vi "TalonFXSet.vi"   [LabVIEW 2023]
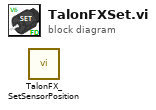
[diagram p0: block diagram]
diagram:
  n1 = call <vilib>:"TalonFX_SetSensorPosition.vi"() -> ()  [unwired: 11 in, 1 out]
